vi "PitchCtrl.vi"(0 "ArrayPairs In":T4={"iStatus"={"Index"=0, "Value"=0.0}, "TIME"={"Index"=1, "Value"=0.0}, "DT"={"Index"=2, "Value"=0.0}, "Blade1PitchPos_rad"={"Index"=3, "Value"=0.0}, "VS_MECHGENPWR"={"Index"=13, "Value"=0.0}, "VS_GENPWR"={"Index"=14, "Value"=0.0}, "GEN_SPEED"={"Index"=19, "Value"=0.0}, "ROTOR_SPEED"={"Index"=20, "Value"=0.0}, "GENTQMEAS"={"Index"=22, "Value"=0.0}, "Y_M"={"Index"=23, "Value"=0.0}, "HORWINDV"={"Index"=26, "Value"=0.0}, "ROOTMOOP1"={"Index"=29, "Value"=0.0}, "ROOTMOOP2"={"Index"=30, "Value"=0.0}, "Blade2PitchPos_rad"={"Index"=32, "Value"=0.0}, "Blade3PitchPos_rad"={"Index"=33, "Value"=0.0}, "ROOTMOOP3"={"Index"=31, "Value"=0.0}, "AVCMSG_SIZE"={"Index"=48, "Value"=0.0}, "INFILE_SIZE "={"Index"=49, "Value"=0.0}, "OUTFILE_SIZE "={"Index"=50, "Value"=0.0}, "FA_ACC"={"Index"=52, "Value"=0.0}, "NUM_BLADES"={"Index"=60, "Value"=0.0}, "BladePitchSetpoint_rad"={"Index"=44, "Value"=0.0}, "TorqueSetpoint_Nm"={"Index"=46, "Value"=0.0}, "OUT_AEROTQ"={"Index"=89, "Value"=0.0}, "Out.RotSpeed "={"Index"=92, "Value"=0.0}, "Out.DEBUG"={"Index"=93, "Value"=0.0}}, 1 "IO Signals In":T6, 3 "ROSCO Params in":T7, 5 "error in (no error)":errorcluster, 6 "PitchCtrl":T2={"P-Gain"=0.0, "Blade pitch operating mode"=enum."From File", "Constant setpoint (deg)"=0.0, "I-Gain"=0.0, "Pitch from File (deg)"=0.0, "Homing vel (rpm)"=0.0, "Max vel (rpm)"=0.0, "Max vel change (rpm/min)"=0.0}, 7 "Time (s)":dbl, 8 "PitchAxis1State":T1, 10 "PitchAxis2State":T1, 12 "PitchAxis3State":T1) -> (13 "Pitch setpoint (rad)":dbl, 14 "ArrayPairs Out":T4={"iStatus"={"Index"=0, "Value"=0.0}, "TIME"={"Index"=1, "Value"=0.0}, "DT"={"Index"=2, "Value"=0.0}, "Blade1PitchPos_rad"={"Index"=3, "Value"=0.0}, "VS_MECHGENPWR"={"Index"=13, "Value"=0.0}, "VS_GENPWR"={"Index"=14, "Value"=0.0}, "GEN_SPEED"={"Index"=19, "Value"=0.0}, "ROTOR_SPEED"={"Index"=20, "Value"=0.0}, "GENTQMEAS"={"Index"=22, "Value"=0.0}, "Y_M"={"Index"=23, "Value"=0.0}, "HORWINDV"={"Index"=26, "Value"=0.0}, "ROOTMOOP1"={"Index"=29, "Value"=0.0}, "ROOTMOOP2"={"Index"=30, "Value"=0.0}, "Blade2PitchPos_rad"={"Index"=32, "Value"=0.0}, "Blade3PitchPos_rad"={"Index"=33, "Value"=0.0}, "ROOTMOOP3"={"Index"=31, "Value"=0.0}, "AVCMSG_SIZE"={"Index"=48, "Value"=0.0}, "INFILE_SIZE "={"Index"=49, "Value"=0.0}, "OUTFILE_SIZE "={"Index"=50, "Value"=0.0}, "FA_ACC"={"Index"=52, "Value"=0.0}, "NUM_BLADES"={"Index"=60, "Value"=0.0}, "BladePitchSetpoint_rad"={"Index"=44, "Value"=0.0}, "TorqueSetpoint_Nm"={"Index"=46, "Value"=0.0}, "OUT_AEROTQ"={"Index"=89, "Value"=0.0}, "Out.RotSpeed "={"Index"=92, "Value"=0.0}, "Out.DEBUG"={"Index"=93, "Value"=0.0}}, 15 "IO Signals Out":T6, 17 "ROSCO Params Out":T7, 19 "error out":errorcluster)   [LabVIEW 2018]
uses:
  Clusters/RoscoParams.ctl
  Clusters/IOSignals.ctl
  Clusters/ArrayPairs.ctl
  Clusters/SwapArrayCluster.ctl
  Clusters/PitchCtrl.ctl
  Clusters/BladePitchMode.ctl
  Clusters/ElmoState.ctl
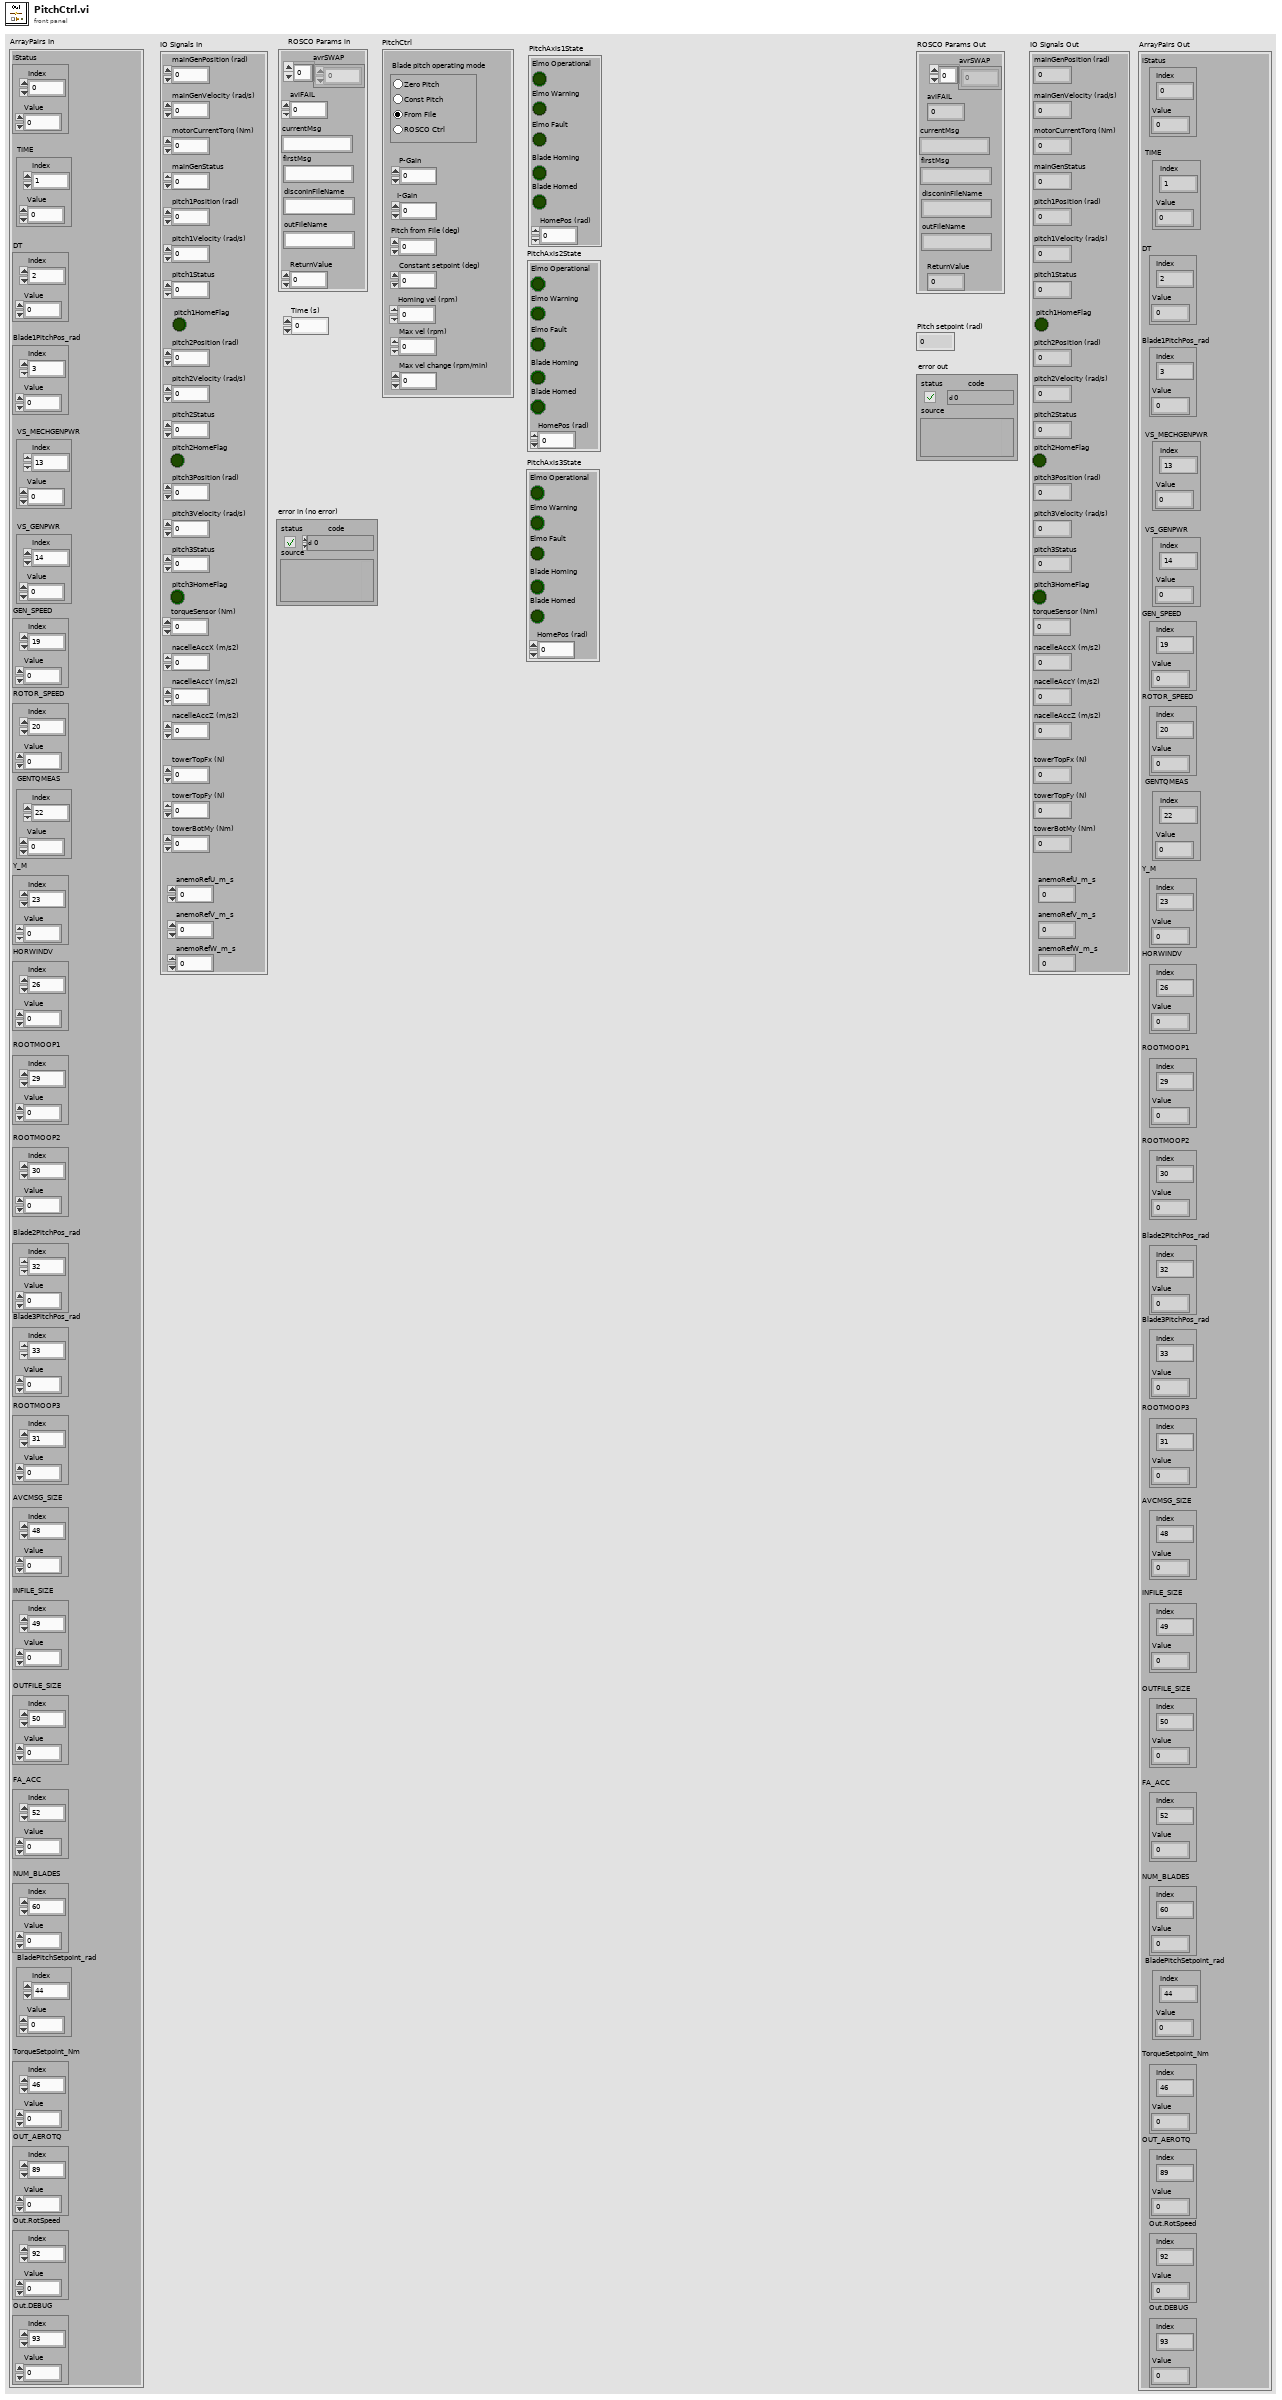
[diagram p1: front panel]
types:
  T1 = typedef "ElmoState.ctl" = cluster{"Elmo Operational":bool, "Elmo Warning":bool, "Elmo Fault":bool, "Blade Homed":bool, "Blade Homing":bool, "HomePos (rad)":dbl}
  T2 = typedef "PitchCtrl.ctl" = cluster{"P-Gain":dbl, "Blade pitch operating mode":T3, "Constant setpoint (deg)":dbl, "I-Gain":dbl, "Pitch from File (deg)":dbl, "Homing vel (rpm)":dbl, "Max vel (rpm)":dbl, "Max vel change (rpm/min)":dbl}
  T3 = typedef "BladePitchMode.ctl" = enum32{"Zero pitch", "Const pitch", "From File", "ROSCO Ctrl"}
  T4 = typedef "ArrayPairs.ctl" = cluster{"iStatus":T5, "TIME":T5, "DT":T5, "Blade1PitchPos_rad":T5, "VS_MECHGENPWR":T5, "VS_GENPWR":T5, "GEN_SPEED":T5, "ROTOR_SPEED":T5, "GENTQMEAS":T5, "Y_M":T5, "HORWINDV":T5, "ROOTMOOP1":T5, "ROOTMOOP2":T5, "Blade2PitchPos_rad":T5, "Blade3PitchPos_rad":T5, "ROOTMOOP3":T5, "AVCMSG_SIZE":T5, "INFILE_SIZE ":T5, "OUTFILE_SIZE ":T5, "FA_ACC":T5, "NUM_BLADES":T5, "BladePitchSetpoint_rad":T5, "TorqueSetpoint_Nm":T5, "OUT_AEROTQ":T5, "Out.RotSpeed ":T5, "Out.DEBUG":T5}
  T5 = typedef "SwapArrayCluster.ctl" = cluster{"Index":i32, "Value":dbl}
  T6 = typedef "IOSignals.ctl" = cluster{"mainGenPosition (rad)":dbl, "motorCurrentTorq (Nm)":dbl, "mainGenVelocity (rad/s)":dbl, "mainGenStatus":u16, "pitch1Position (rad)":dbl, "pitch1Velocity (rad/s)":dbl, "pitch1Status":u16, "pitch2Position (rad)":dbl, "pitch2Velocity (rad/s)":dbl, "pitch2Status":u16, "pitch3Position (rad)":dbl, "pitch3Velocity (rad/s)":dbl, "pitch3Status":u16, "torqueSensor (Nm)":dbl, "nacelleAccX (m/s2)":dbl, "nacelleAccY (m/s2)":dbl, "nacelleAccZ (m/s2)":dbl, "pitch1HomeFlag":bool, "pitch2HomeFlag":bool, "pitch3HomeFlag":bool, "towerTopFx (N)":dbl, "towerTopFy (N)":dbl, "towerBotMy (Nm)":dbl, "anemoRefU_m_s":dbl, "anemoRefV_m_s":dbl, "anemoRefW_m_s":dbl}
  T7 = typedef "RoscoParams.ctl" = cluster{"avrSWAP":dbl[], "aviFAIL":i32, "currentMsg":string, "ReturnValue":i32, "disconInFileName":string, "outFileName":string, "firstMsg":string}
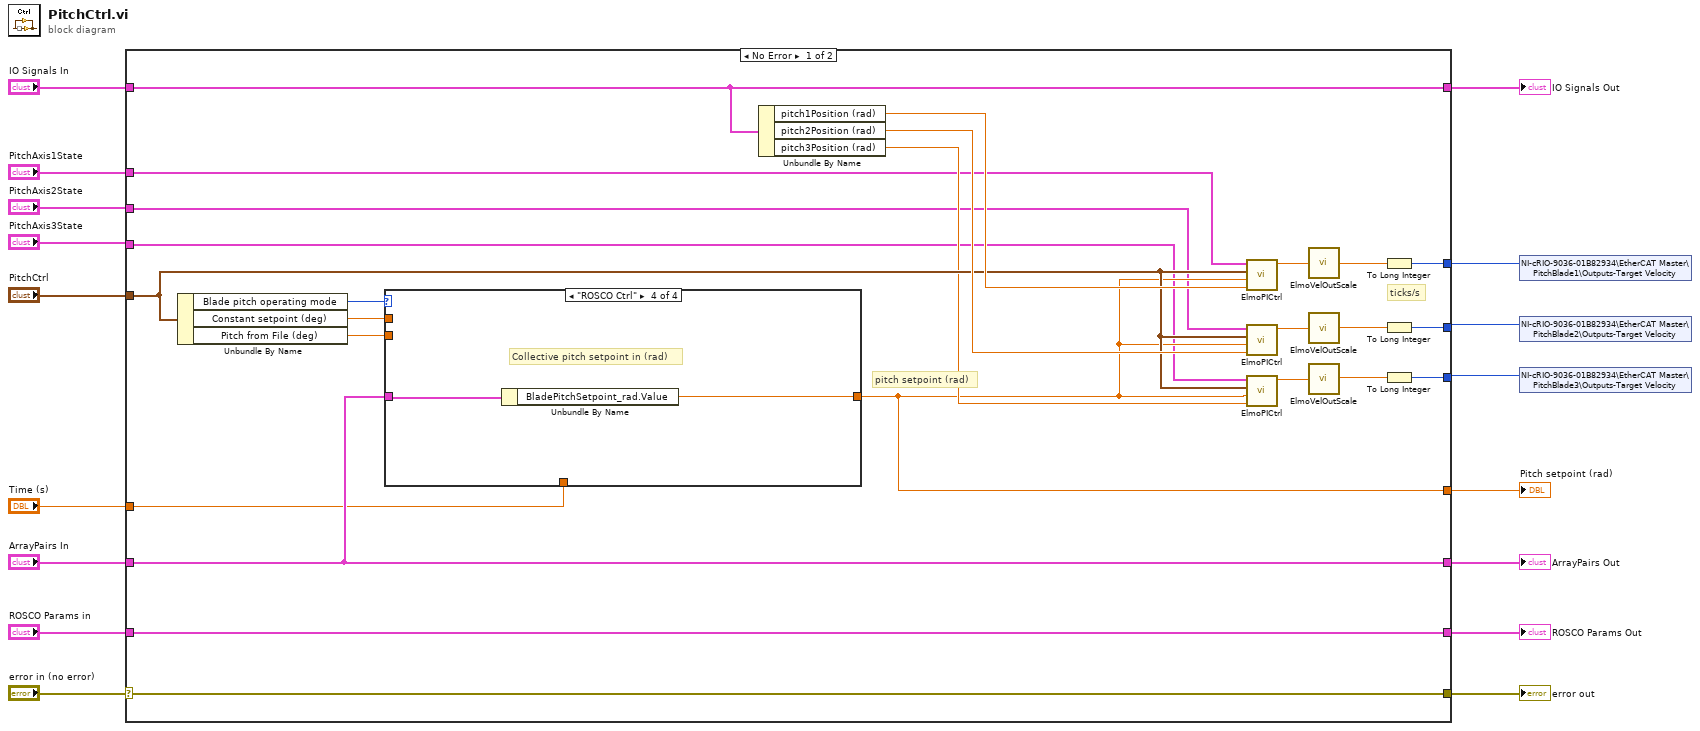
[diagram p0: block diagram]
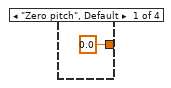
[diagram p2: hidden frame]
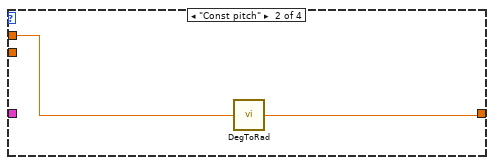
[diagram p3: hidden frame]
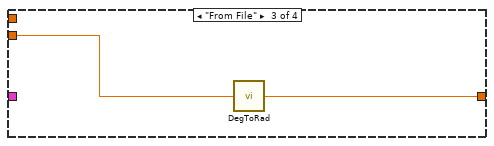
[diagram p4: hidden frame]
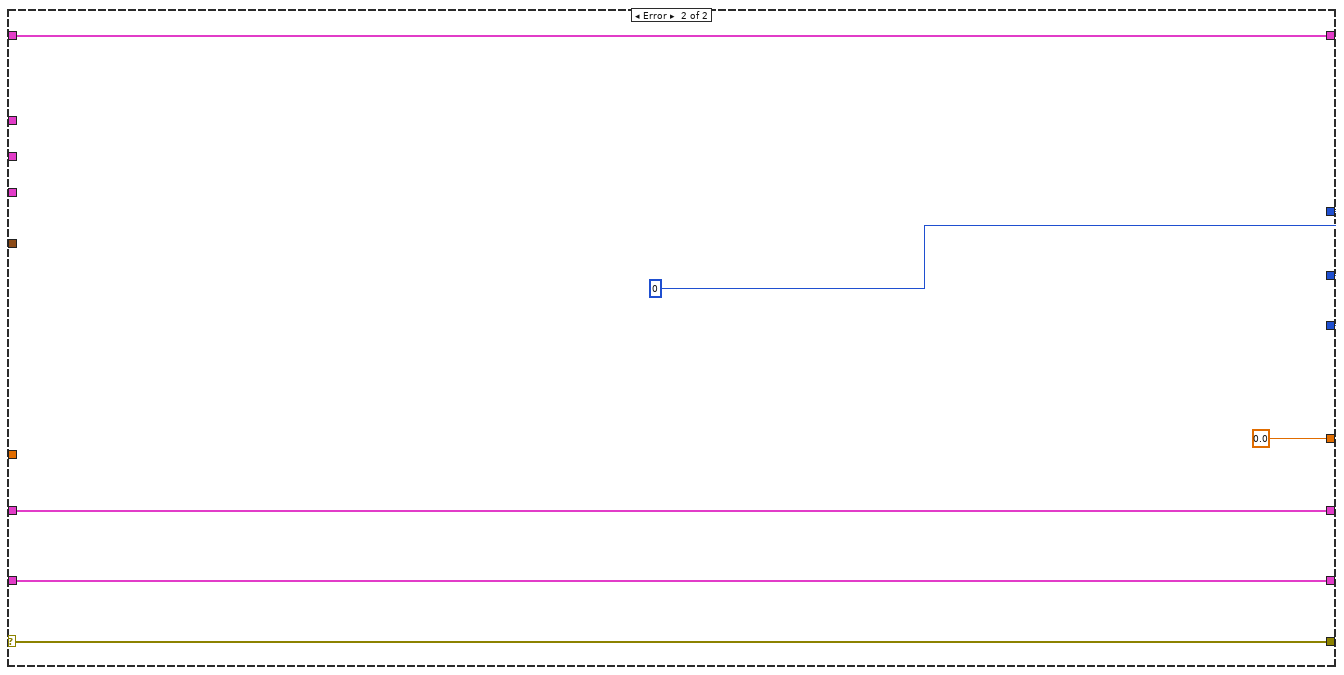
[diagram p5: hidden frame]
diagram:
  n1 = case shown="No Error" "error in (no error)" {
    selector: "error in (no error)" -> [w42 w55]
    tunnel: [w42 w55] -> w16
    tunnel: [w41 w54] -> w14
    tunnel: "ROSCO Params in" -> [w41 w54]
    tunnel: [w40 w53] -> w12
    tunnel: "ArrayPairs In" -> [w40 w53]
    tunnel: [w39 w52] -> w10
    tunnel: "IO Signals In" -> [w39 w52]
    tunnel: [w38 w51] -> w4
    tunnel: [w34 w51] -> w6
    tunnel: [w33 w51] -> w5
    tunnel: "PitchCtrl" -> [w28 _]
    tunnel: "Time (s)" -> [w31 _]
    tunnel: [w23 0.0 ("Value")] -> w8
    tunnel: "PitchAxis3State" -> [w20 _]
    tunnel: "PitchAxis2State" -> [w19 _]
    tunnel: "PitchAxis1State" -> [w18 _]
    frame No Error {
      # "pitch setpoint (rad)"
      # "ticks/s"
      n2 = Unbundle By Name(w28) -> ("Blade pitch operating mode"=w21:T3, "Constant setpoint (deg)"=w32:dbl, "Pitch from File (deg)"=w22:dbl)
      n3 = case shown="\"ROSCO Ctrl\"" w21 {
        tunnel: w40 -> [_ _ _ w49]
        tunnel: [0.0 ("rad") w44 w47 w48] -> w23
        tunnel: w32 -> [_ w45 _ _]
        tunnel: w31 -> [_ _ _ _]
        tunnel: w22 -> [_ _ w46 _]
        frame "Zero pitch", Default {
        }
        frame "Const pitch" {
          n4 = call "DegToRad.vi"("deg"=w45) -> ("rad"=w44:dbl)
        }
        frame "From File" {
          n5 = call "DegToRad.vi"("deg"=w46) -> ("rad"=w47:dbl)
        }
        frame "ROSCO Ctrl" {
          # "Collective pitch setpoint in (rad)"
          n6 = Unbundle By Name(w49) -> ("BladePitchSetpoint_rad.Value"=w48:dbl)
        }
      }
      n7 = Unbundle By Name(w39) -> ("pitch1Position (rad)"=w30:dbl, "pitch2Position (rad)"=w29:dbl, "pitch3Position (rad)"=w27:dbl)
      n8 = call "ElmoPICtrl.vi"("Actual pitch angle (rad)"=w30, "Pitch setpoint (rad)"=w23, "Pitch Ctrl"=w28, "PitchAxis1State"=w18) -> ("Demand out (rad/s)"=w26:dbl)  [unwired: 7 in]
      n9 = call "ElmoPICtrl.vi"("Actual pitch angle (rad)"=w29, "Pitch setpoint (rad)"=w23, "Pitch Ctrl"=w28, "PitchAxis1State"=w19) -> ("Demand out (rad/s)"=w25:dbl)  [unwired: 7 in]
      n10 = call "ElmoPICtrl.vi"("Actual pitch angle (rad)"=w27, "Pitch setpoint (rad)"=w23, "Pitch Ctrl"=w28, "PitchAxis1State"=w20) -> ("Demand out (rad/s)"=w24:dbl)  [unwired: 7 in]
      n11 = call "ElmoVelOutScale.vi"("vel (rad/s)"=w26) -> ("vel (tick/s)"=w37:dbl)
      n12 = call "ElmoVelOutScale.vi"("vel (rad/s)"=w25) -> ("vel (tick/s)"=w36:dbl)
      n13 = call "ElmoVelOutScale.vi"("vel (rad/s)"=w24) -> ("vel (tick/s)"=w35:dbl)
      n14 = To Long Integer(number=w37) -> (32bit integer=w38:i32)
      n15 = To Long Integer(number=w36) -> (32bit integer=w34:i32)
      n16 = To Long Integer(number=w35) -> (32bit integer=w33:i32)
    }
    frame Error {
      w51 = 0
    }
  }
  "error out" <- w16
  "ROSCO Params Out" <- w14
  "IO Signals Out" <- w10
  "ArrayPairs Out" <- w12
  "Pitch setpoint (rad)" <- w8
  n17 = shared-variable "NI-cRIO-9036-01B82934\\EtherCAT Master\\PitchBlade1\\Outputs-Target Velocity"(w4) -> ()  [unwired: 1 in, 1 out]
  n18 = shared-variable "NI-cRIO-9036-01B82934\\EtherCAT Master\\PitchBlade2\\Outputs-Target Velocity"(w6) -> ()  [unwired: 1 in, 1 out]
  n19 = shared-variable "NI-cRIO-9036-01B82934\\EtherCAT Master\\PitchBlade3\\Outputs-Target Velocity"(w5) -> ()  [unwired: 1 in, 1 out]
